vi "Task Self Running.vi"(8 "error in (no error)":errorcluster, 10 "Message In":refnum<class "Message.lvclass">, 11 "System Actor in":refnum<class "System Actor.lvclass">) -> (0 "error out":errorcluster, 3 "System Actor out":refnum<class "System Actor.lvclass">)   [LabVIEW 2024, in "System Actor.lvclass"]
uses:
  System Actor.lvclass
  Message/Message.lvclass
  Message/Message.lvclass/Message.ctl
  Message/Public Data/Read Single Task.vi
  Task/Task Ancestor/Task Ancestor.lvclass
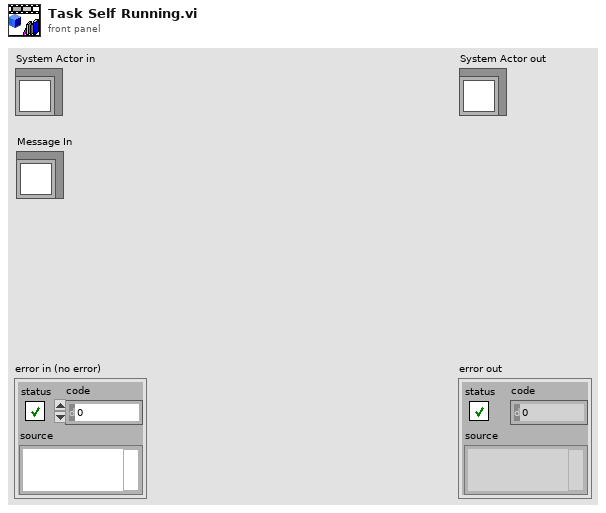
[diagram p1: front panel]
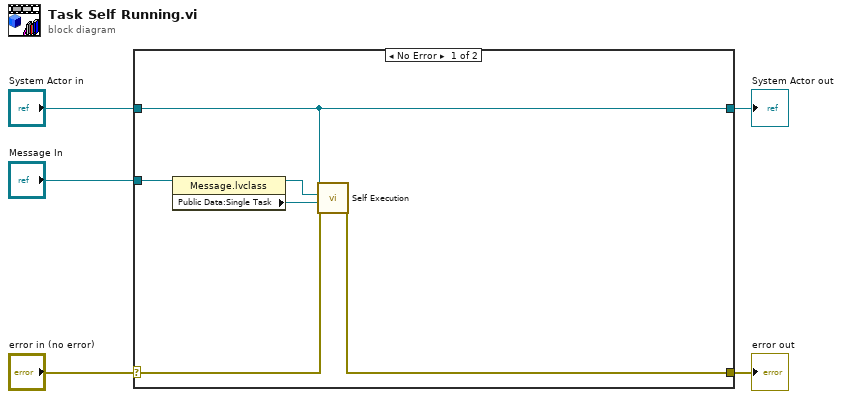
[diagram p0: block diagram]
diagram:
  n1 = case shown="No Error" "error in (no error)" {
    selector: "error in (no error)" -> [w7 w13]
    tunnel: [w6 w13] -> w4
    tunnel: [w8 w12] -> w2
    tunnel: "System Actor in" -> [w8 w12]
    tunnel: "Message In" -> [w11 _]
    frame No Error {
      n2 = property class="Message.lvclass"(reference=w11) -> (reference out=w9:refnum<class "Message.lvclass">, "Public Data:Single Task"=w10:refnum<class "Task Ancestor.lvclass">)  [unwired: 1 in, 1 out]
      n3 = call-dynamic "Self Execution.vi"("error in (no error)"=w7, "Task Ancestor In"=w10, "Message In"=w9, "Actor In"=w8) -> ("error out"=w6:errorcluster)  [unwired: 4 in, 3 out]
    }
    frame Error {
    }
  }
  "error out" <- w4
  "System Actor out" <- w2
